vi "Read.vi"(0 "00-02-9234 Present":bool, 5 "00-03-9402 Present":bool) -> (4 "00-02-9234 AI":fxp<+/-,24,4>[](array[numeric]) format="%.22g", 6 "00-03-9402 DIO":bool[](array[boolean]), 15 "error out":errorcluster)   [LabVIEW 2018]
uses:
  <vilib>/rvi/eio/common/nirviEmuTemplateMethod_errors.vi
  <vilib>/eio/EIONode/EIONode.xnode
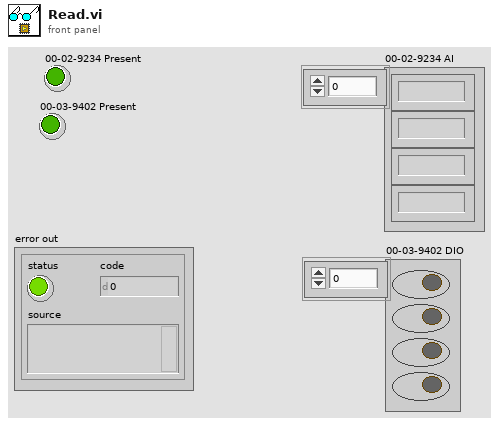
[diagram p1: front panel]
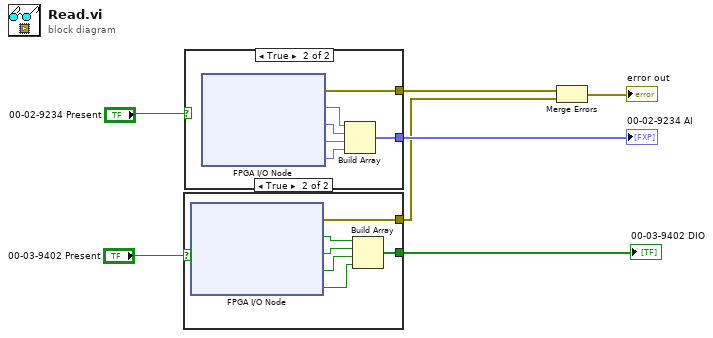
[diagram p0: block diagram]
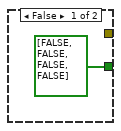
[diagram p2: hidden frame]
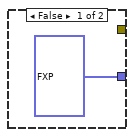
[diagram p3: hidden frame]
diagram:
  n1 = case shown="True" "00-03-9402 Present" {
    tunnel: [bool[] [FALSE, FALSE, FALSE, FALSE] w14] -> w6
    tunnel: [_ w9] -> w1
    frame False {
    }
    frame True {
      n2 = xnode "FPGA I/O Node"() -> ("error out"=w9:errorcluster, "00-03-9402/DIO0"=w13:bool, "00-03-9402/DIO1"=w12:bool, "00-03-9402/DIO2"=w11:bool, "00-03-9402/DIO3"=w10:bool)  [unwired: 5 in, 4 out]
      n3 = Build Array(w13, w12, w11, w10) -> (w14:bool[])
    }
  }
  "00-03-9402 DIO" <- w6
  n4 = case shown="True" "00-02-9234 Present" {
    tunnel: [fxp<+/-,24,4>[] [0.0, 0.0, 0.0, 0.0] w21] -> w7
    tunnel: [_ w16] -> w2
    frame False {
    }
    frame True {
      n5 = xnode "FPGA I/O Node"() -> ("error out"=w16:errorcluster, "00-02-9234/AI0"=w17:fxp<+/-,24,4>, "00-02-9234/AI1"=w18:fxp<+/-,24,4>, "00-02-9234/AI2"=w19:fxp<+/-,24,4>, "00-02-9234/AI3"=w20:fxp<+/-,24,4>)  [unwired: 5 in, 4 out]
      n6 = Build Array(w17, w18, w19, w20) -> (w21:fxp<+/-,24,4>[])
    }
  }
  "00-02-9234 AI" <- w7
  n7 = Merge Errors(w2, w1) -> (→"error out":errorcluster)
